vi "Send Receive.vi"   [LabVIEW 2021, in "Simple VISA Reader Driver.lvclass"]
uses:
  Simple VISA Reader/Simple VISA Reader Driver.lvclass
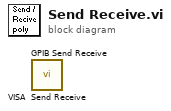
[diagram p0: block diagram]
diagram:
  n1 = call "VISA  Send Receive.vi"() -> ()  [unwired: 9 in, 3 out]
  n2 = call "GPIB Send Receive.vi"() -> ()  [unwired: 9 in, 3 out]
